vi "printed picture.vi"() -> ()   [LabVIEW 2016]
panel:
  out "XY Graph":cluster{i32, i32}[](graph)
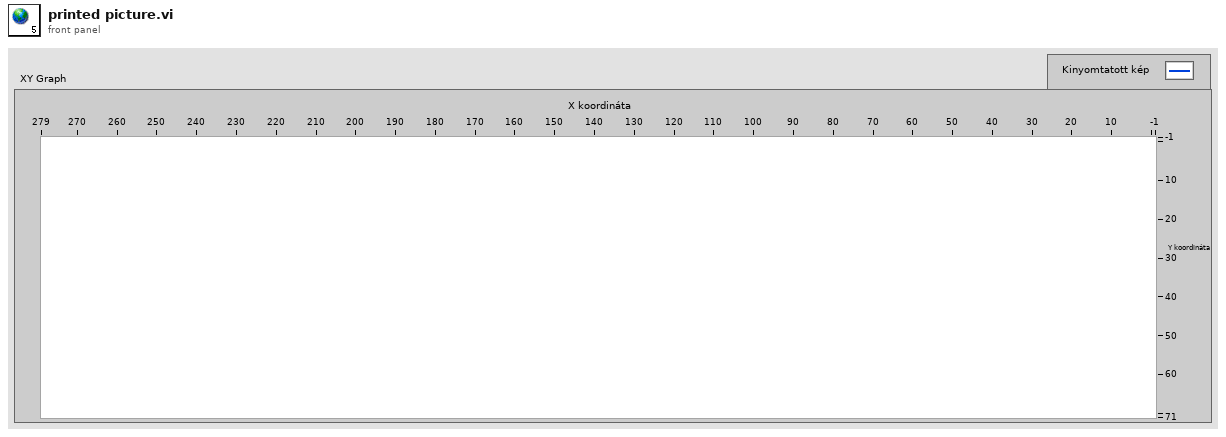
[diagram p1: front panel]
diagram:
